vi "JSONrpc-Example.vi"(8 "error in (no error)":errorcluster) -> (0 "error out":errorcluster)   [LabVIEW 2019]
uses:
  <vilib>/numeric/Random Number (Range) DBL.vi
  <vilib>/numeric/Random Number (Range) U64.vi
  4c12f335-3af6-49f5-9257-0130b4f6318c.vi
  e861ad0b-bed5-4796-b07d-8449c8f87c08.vi
  <vilib>/numeric/sub_Random U32.vi
  4c12f335-3af6-49f5-9257-0130b4f6318c.vi/7b8b0f69-2f54-4be0-9abe-caa8645179b0.vi
  4c12f335-3af6-49f5-9257-0130b4f6318c.vi/307d6119-f25b-468d-b3e0-ef9f1a1a6fd2.vi
  e861ad0b-bed5-4796-b07d-8449c8f87c08.vi/dab2e044-56e2-4a2a-97c6-8deb14d6665e.vi
  e861ad0b-bed5-4796-b07d-8449c8f87c08.vi/55732a74-c736-46f3-938e-d0df42ffec67.vi
  <vilib>/Utility/Data Type/Get Type Information.vi
  <vilib>/JDP Science/JSONtext/JSON text to Variant.vi
  <vilib>/JDP Science/JSONtext/LVClass Serializer/JSONtext LVClass Serializer.lvclass
  JSON-RPC.lvlib
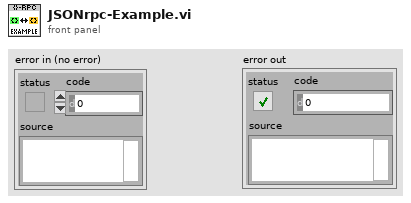
[diagram p1: front panel]
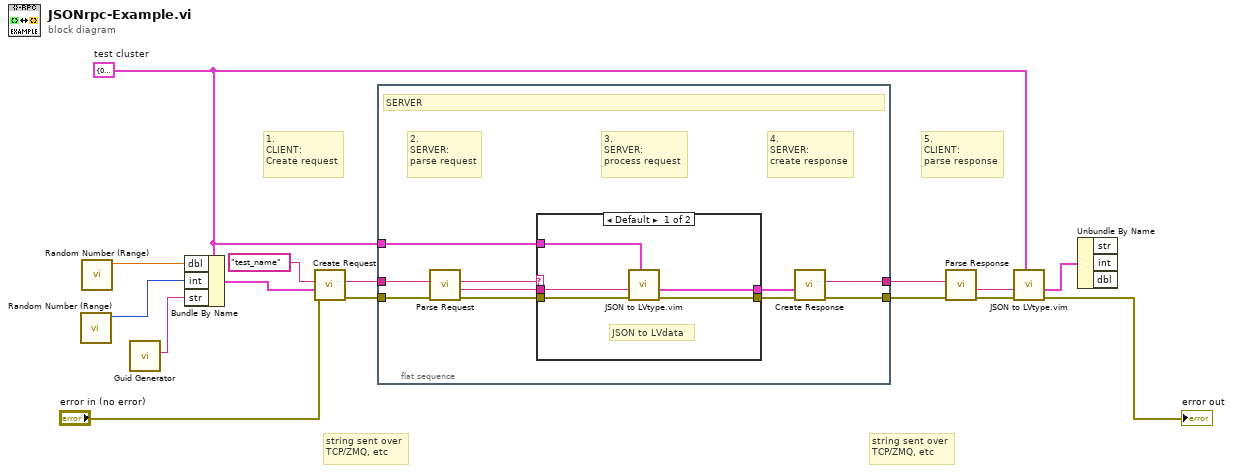
[diagram p0: block diagram]
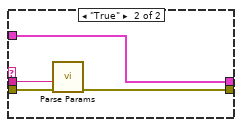
[diagram p2: hidden frame]
diagram:
  w7 = cluster{"dbl":dbl, "int":i32, "str":string} {"dbl"=0.0, "int"=0, "str"=""}  # test cluster
  # "string sent over\nTCP/ZMQ, etc"
  # "string sent over\nTCP/ZMQ, etc"
  # "5.\nCLIENT:\nparse response"
  # "1.\nCLIENT:\nCreate request"
  n1 = call-poly <vilib>:"Random Number (Range).vi"() -> ("number"=w11:u64)  [unwired: 11 in]
  n2 = call-poly <vilib>:"Random Number (Range).vi"() -> ("number"=w10:dbl)  [unwired: 11 in]
  n3 = call <vilib>:"Guid Generator.vi"() -> ("GUID"=w9:string)  [unwired: 10 in, 1 out]
  n4 = Bundle By Name(cluster=w7, "dbl"=w10, "int"=w11, "str"=w9) -> (w5:cluster{"dbl":dbl, "int":i32, "str":string})
  n5 = call "Create Request.vi"("error in (no error)"="error in (no error)", "params"=w5, "method"="test_name") -> ("error out"=w14:errorcluster, "<JSON> Requests"=w15:string)  [unwired: 6 in, 1 out]
  n6 = flat-sequence {
    tunnel: w15 -> [w25]
    tunnel: w14 -> [w21]
    tunnel: [w20] -> w13
    tunnel: [w19] -> w12
    tunnel: w7 -> [w17]
    frame #0 {
      # "2.\nSERVER:\nparse request"
      # "3.\nSERVER:\nprocess request"
      # "4.\nSERVER:\ncreate response"
      # "SERVER"
      n7 = call "Parse Request.vi"("error in (no error)"=w21, "<JSON> Requests"=w25) -> ("error out"=w22:errorcluster, "Params"=w23:string, "Methods"=w24:string)  [unwired: 6 in, 1 out]
      n8 = case shown="Default" w24 {
        tunnel: w23 -> [w27 w34]
        tunnel: w22 -> [w30 w33]
        tunnel: [w29 w32] -> w18
        tunnel: w17 -> [w28 w31]
        tunnel: [w26 w31] -> w16
        frame Default {
          # "JSON to LVdata"
          n9 = call "JSON to LVtype.vim"("type"=w28, "error in (no error)"=w30, "JSON Data in"=w27) -> ("error out"=w29:errorcluster, "Data out"=w26:cluster{"dbl":dbl, "int":i32, "str":string})  [unwired: 7 in]
        }
        frame "True" {
          n10 = call "Parse Params.vi"("error in (no error)"=w33, "<JSON> Params"=w34) -> ("error out"=w32:errorcluster)  [unwired: 7 in, 2 out]
        }
      }
      n11 = call "Create Response.vi"("error in (no error)"=w18, "result"=w16) -> ("error out"=w19:errorcluster, "<JSON> Response"=w20:string)  [unwired: 8 in]
    }
  }
  n12 = call "Parse Response.vi"("error in (no error)"=w12, "<JSON> Response"=w13) -> ("error out"=w8:errorcluster, "results"=w3:string)  [unwired: 7 in, 1 out]
  n13 = call "JSON to LVtype.vim"("type"=w7, "error in (no error)"=w8, "JSON Data in"=w3) -> ("error out"=→"error out":errorcluster, "Data out"=w2:cluster{"dbl":dbl, "int":i32, "str":string})  [unwired: 7 in]
  n14 = Unbundle By Name(w2) -> ()  [unwired: 3 out]
